vi "Save VI.vi"(8 "error in (no error)":errorcluster, 11 "Assert VI Path":path) -> (0 "error out":errorcluster)   [LabVIEW 2016]
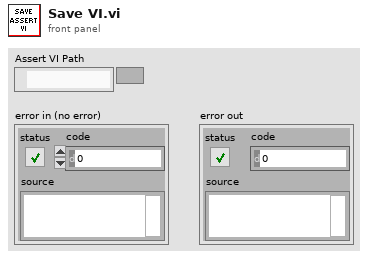
[diagram p1: front panel]
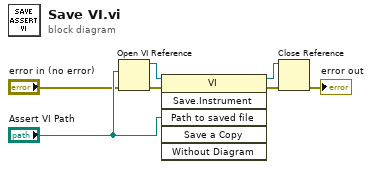
[diagram p0: block diagram]
diagram:
  n1 = Open VI Reference(vi path="Assert VI Path", error in (no error)="error in (no error)") -> (vi reference=w5:refnum<vi>, error out=w2:errorcluster)  [unwired: 4 in]
  n2 = invoke class="VI" method="Save.Instrument"(reference=w5, error in=w2, "Path to saved file"="Assert VI Path") -> (reference out=w6:refnum<vi>, error out=w3:errorcluster)  [unwired: 3 in, 4 out]
  n3 = Close Reference(reference=w6, error in (no error)=w3) -> (error out=→"error out":errorcluster)
